vi "Export Unmapped Channels.vi"(8 "error in (no error)":errorcluster, 9 "Filtered Node":string, 10 "Path":path, 11 "SDF Ref":refnum<k24>) -> (0 "error out":errorcluster)   [LabVIEW 2016, in "System Mapping Tool.lvlib"]
uses:
  System Mapping Tool.lvlib
  NationalInstruments.VeriStand.SystemDefinitionAPI
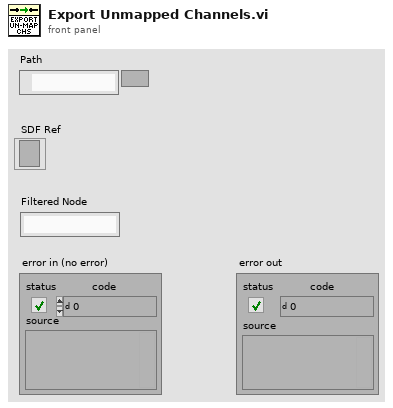
[diagram p1: front panel]
types:
  T1 = enum16{"open", "replace", "create", "open or create", "replace or create", "replace or create with confirmation"}
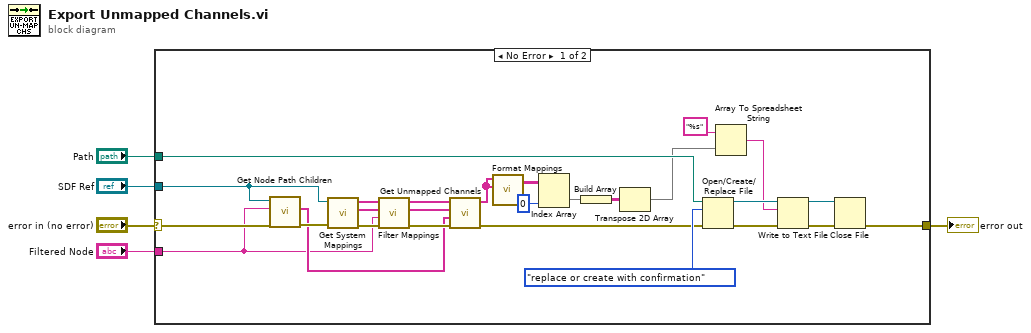
[diagram p0: block diagram]
diagram:
  n1 = case shown="No Error" "error in (no error)" {
    selector: "error in (no error)" -> [w20 w33]
    tunnel: [w25 w33] -> w4
    tunnel: "SDF Ref" -> [w18 _]
    tunnel: "Path" -> [w24 _]
    tunnel: "Filtered Node" -> [w6 _]
    frame No Error {
      n2 = call "Get Node Path Children.vi"("error in (no error)"=w20, "Node Path"=w6, "SDF Ref"=w18) -> ("error out"=w19:errorcluster, "Children"=w13:string[])  [unwired: 7 in]
      n3 = call "Get System Mappings.vi"("error in (no error)"=w19, "SDF Ref"=w18) -> ("error out"=w23:errorcluster, "Destinations"=w21:string[], "Sources"=w22:string[])  [unwired: 7 in]
      n4 = call "Filter Mappings.vi"("error in (no error)"=w23, "Path to Filter"=w6, "Destinations"=w21, "Sources"=w22) -> ("error out"=w17:errorcluster, "Filtered Destinations"=w14:string[], "Filtered Sources"=w15:string[])  [unwired: 5 in]
      n5 = call "Get Unmapped Channels.vi"("error in (no error)"=w17, "All Channels"=w13, "Destinations"=w14, "Sources"=w15) -> ("error out"=w16:errorcluster, "Unmapped Channels"=w8:string[])  [unwired: 6 in]
      n6 = call "Format Mappings.vi"("Destinations"=w8, "Sources"=w8) -> ("Mappings"=w12:string[][])  [unwired: 3 in]
      n7 = Index Array(array=w12, index (col)=0 ("disabled index (col)")) -> (element=w10:string[])  [unwired: 1 in]
      n8 = Build Array(w10) -> (w9:string[][])
      n9 = Transpose 2D Array(2D array=w9) -> (transposed array=w7:string[][])
      n10 = Open/Create/Replace File(file path (use dialog)=w24, error in=w16, operation (0:open)=T1."replace or create with confirmation") -> (refnum out=w30:refnum<file>, error out=w26:errorcluster)  [unwired: 3 in, 1 out]
      n11 = Array To Spreadsheet String(array=w7, 3:"%s" ("format string")) -> (spreadsheet string=w29:string)  [unwired: 1 in]
      n12 = Write to Text File(file (use dialog)=w30, text=w29, error in=w26) -> (refnum out=w27:refnum<file>, error out=w28:errorcluster)  [unwired: 1 in, 1 out]
      n13 = Close File(refnum=w27, error in=w28) -> (error out=w25:errorcluster)  [unwired: 1 out]
    }
    frame Error {
    }
  }
  "error out" <- w4
